vi "StreamInitRT.vi"() -> (0 "data type":T1, 2 "reader buffer size":i32, 3 "reader name":string)   [LabVIEW 2017]
uses:
  TypeDefs/DataStreamCluster.ctl
  TypeDefs/CommandsRT.ctl
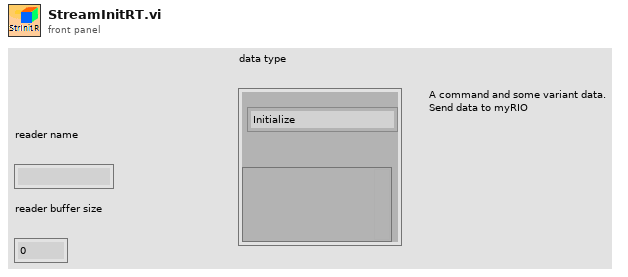
[diagram p1: front panel]
types:
  T1 = typedef "DataStreamCluster.ctl" = cluster{"Commands":T2, "Variant":variant}
  T2 = typedef "CommandsRT.ctl" = enum16{"Initialize", "Turn", "Grip", "Exit"}
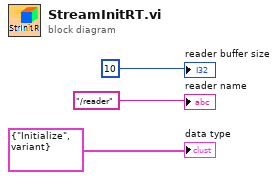
[diagram p0: block diagram]
diagram:
  "reader name" <- "/reader" ("reader name")
  "reader buffer size" <- 10 ("reader buffer size")
  "data type" <- T1 {"Commands"=enum."Initialize", "Variant"=variant} ("output cluster")
